vi "HEUI.vi"(0 "LED Update Rate (s)":dbl=0.25 caption="Delay Time (s)", 6 "HEUI_Buttons":T1, 7 "stop":bool, 11 "Error In":errorcluster) -> (5 "HEUI_LEDs":T2, 15 "Error Out":errorcluster)   [LabVIEW 2014]
doc: "This VI controls the high end 2015 VA washer UI board. The VI updates the status of the LEDs every 'LED update rate (s)' number of seconds. The VI allows the user to press buttons and select a cycle."
uses:
  type defs/HEUI_Buttons.ctl
  type defs/HEUI_LEDs.ctl
  Utility/Labview GEA2 Toolkit v2.1/type defs/Data In.ctl
  Utility/Labview GEA2 Toolkit v2.1/type defs/Source_Destination.ctl
  Utility/Labview GEA2 Toolkit v2.1/type defs/ERD Read Data In.ctl
  Utility/Labview GEA2 Toolkit v2.1/type defs/ERD Write Data In.ctl
  type defs/HEUI Switches.ctl
  Utility/Labview GEA2 Toolkit v2.1/library/GEA2_Toolkit.lvlib
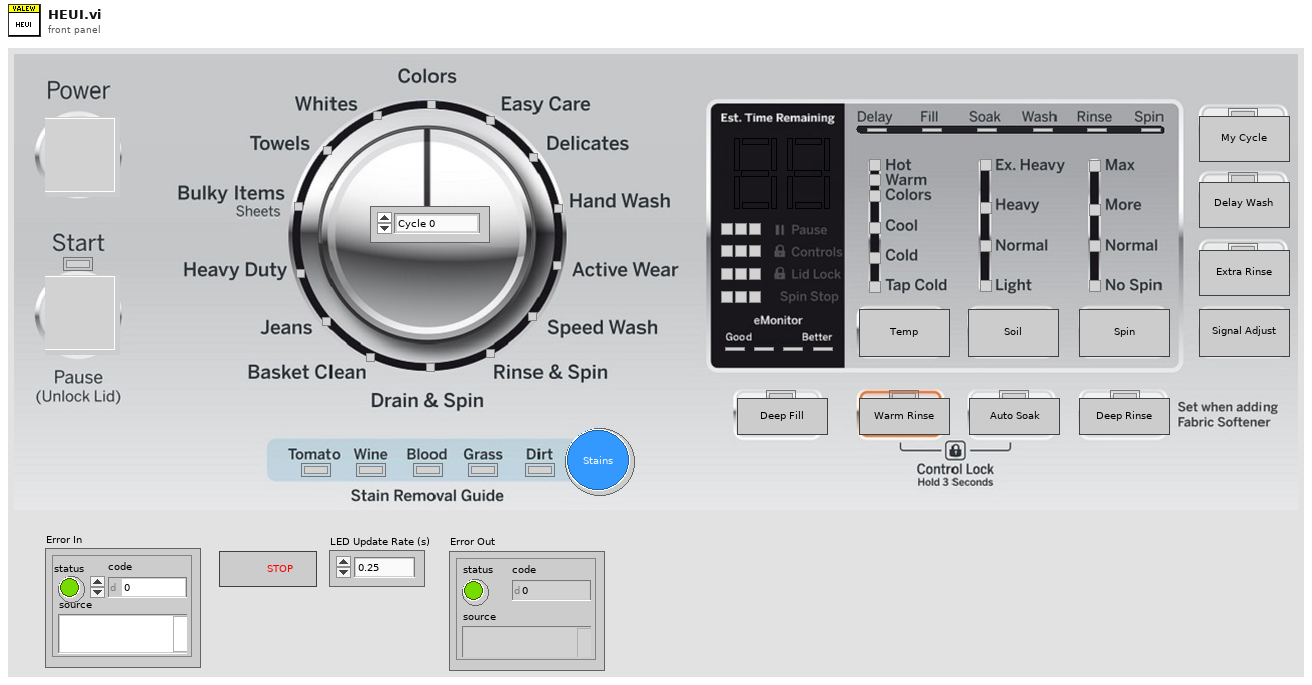
[diagram p1: front panel]
types:
  T1 = typedef "HEUI_Buttons.ctl" = cluster{"SW204 - Signal Adjust":bool, "SW203 - Extra Rinse":bool, "SW201 - My Cycle":bool, "SW202 - Delay Wash":bool, "SW211 - Deep Fill":bool, "SW210 - Warm Rinse":bool, "SW208 - Auto Soak":bool, "SW206 - Deep Rinse":bool, "SW209 - Temp":bool, "SW207 - Soil":bool, "SW205 - Spin":bool, "SW212 - Stains":bool, "Cycle Selection":enum16{"Cycle 0", "Cycle 1", "Cycle 2", "Cycle 3", "Cycle 4", "Cycle 5", "Cycle 6", "Cycle 7", "Cycle 8", "Cycle 9", "Cycle 10", "Cycle 11", "Cycle 12", "Cycle 13"}, "SW213 - Power":bool, "SW214 - Start/Pause":bool}
  T2 = typedef "HEUI_LEDs.ctl" = cluster{"Z101 - Start":bool, "Z103 - Colors":bool, "Z104 - Whites":bool, "Z105 - Towels":bool, "Z106 - Bulky Items":bool, "Z107 - Heavy Duty":bool, "Z108 - Jeans":bool, "Z109 - Basket Clean":bool, "Z110 - Drain and Spin":bool, "Z111 - Rinse and Spin":bool, "Z112 - Speed Wash":bool, "Z113 - Active Wear":bool, "Z114 - Hand Wash":bool, "Z115 - Delicates":bool, "Z116 - Easy Care":bool, "Z117 - Tomato":bool, "Z118 - Wine":bool, "Z119 - Blood":bool, "Z120 - Grass":bool, "Z121 - Dirt":bool, "Z122_MSB_A":bool, "Z123_MSB_B":bool, "Z124_MSB_G":bool, "Z125_MSB_C":bool, "Z126_MSB_D":bool, "Z127_MSB_E":bool, "Z128_MSB_F":bool, "Z129_LSB_A":bool, "Z130_LSB_B":bool, "Z131_LSB_G":bool, "Z132_LSB_C":bool, "Z133_LSB_D":bool, "Z134_LSB_E":bool, "Z135_LSB_F":bool, "Z136 - Pause":bool, "Z137 - Pause":bool, "Z138 - Lock Controls":bool, "Z139 - Lock Controls":bool, "Z140 - Lock Controls":bool, "Z141 - Lid Lock":bool, "Z142 - Lid Lock":bool, "Z143 - Lid Lock":bool, "Z144 - Good":bool, "Z145":bool, "Z146":bool, "Z147 - Better":bool, "Z148 - Delay":bool, "Z149 - Fill":bool, "Z150 - Soak":bool, "Z151 - Wash":bool, "Z152 - Rinse":bool, "Z153 - Spin":bool, "Z154 - Hot":bool, "Z155 - Warm":bool, "Z156 - Colors":bool, "Z157 - Cool":bool, "Z158 - Cold":bool, "Z159 - Tap Cold":bool, "Z160 - Extra Heavy":bool, "Z161 - Heavy":bool, "Z162 - Normal":bool, "Z163 - Light":bool, "Z164 - Max Spin":bool, "Z165 - More Spin":bool, "Z166 - Normal Spin":bool, "Z167 - No Spin":bool, "Z168 - Extra Rinse":bool, "Z170 - Deep Rinse":bool, "Z171 - Auto Soak":bool, "Z172 - Warm Rinse":bool, "Z173 - Deep Fill":bool, "Z174 - My Cycles":bool, "Z175 - Delay Wash":bool, "Z176 - Spin Stop":bool, "Z177 - Spin Stop":bool, "Z178 - Spin Stop":bool, "Z179 - Pause":bool, "Z109":bool, "Z110":bool, "Z123":bool, "Z124":bool, "Z140":bool, "Unused0":bool, "Unused1":bool, "Unused2":bool, "Unused3":bool, "Channel_Off":bool, "Channel_Cycle_Unmapped":bool}
  T3 = typedef "GEA2_Toolkit.lvlib/ERD Write Data In.ctl" = cluster{"ERD Number":u16, "Data Type":enum16{"string", "boolean", "uint8_t", "uint16_t", "uint32_t"}, "Data":string}
  T4 = typedef "GEA2_Toolkit.lvlib/ERD Read Data In.ctl" = cluster{"ERD Number":u16, "Data Type":enum16{"string", "boolean", "uint8_t", "uint16_t", "uint32_t", "uint64_t"}}
  T5 = typedef "GEA2_Toolkit.lvlib/Source_Destination.ctl" = cluster{"Source":u8, "Destination":u8}
  T6 = typedef "GEA2_Toolkit.lvlib/Data In.ctl" = cluster{"Source":u8, "Destination":u8, "Command":u8, "Message":string}
  T7 = typedef "HEUI Switches.ctl" = enum16{"Switch Off", "SW201 - My Cycle", "SW202 - Delay Wash", "SW203 - Extra Rinse", "SW204 - Signal Adjust", "SW205 - Spin", "SW206 - Deep Rinse", "SW207 - Soil", "SW208 - Auto Soak", "SW209 - Temp", "SW210 - Warm Rinse", "SW211 - Deep Fill", "SW212 - Stains", "SW213 - Power", "SW214 - Start/Pause", "SW215", "SW216"}
  T8 = enum16{"string", "boolean", "uint8_t", "uint16_t", "uint32_t"}
  T9 = enum16{"Cycle 0", "Cycle 1", "Cycle 2", "Cycle 3", "Cycle 4", "Cycle 5", "Cycle 6", "Cycle 7", "Cycle 8", "Cycle 9", "Cycle 10", "Cycle 11", "Cycle 12", "Cycle 13"}
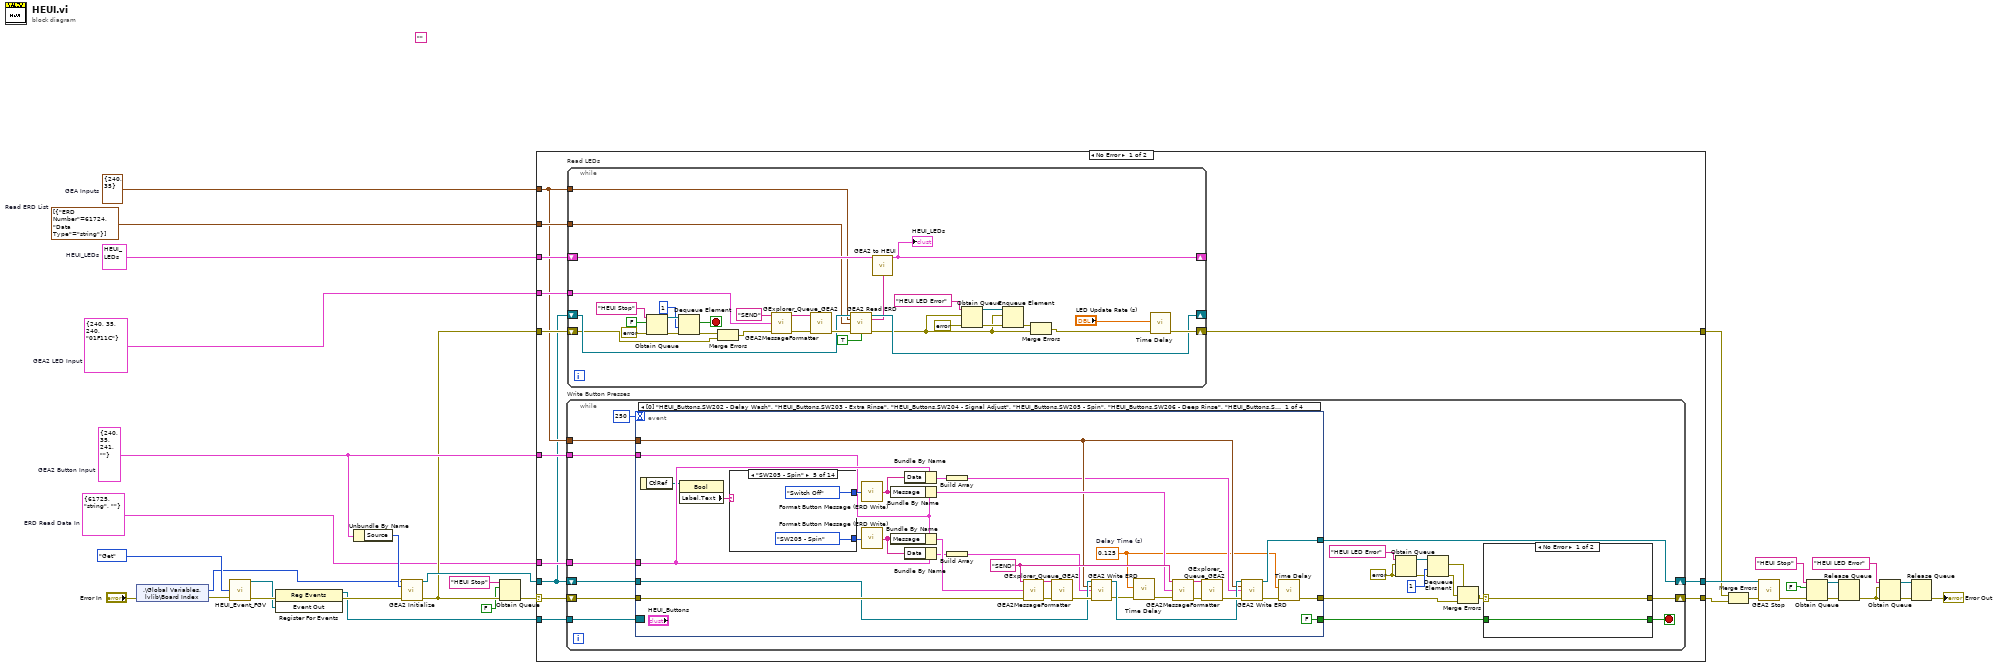
[diagram p0: block diagram]
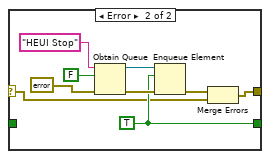
[diagram p2: hidden frame]
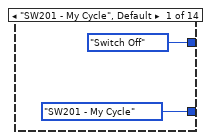
[diagram p3: hidden frame]
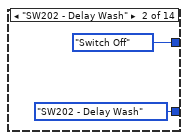
[diagram p4: hidden frame]
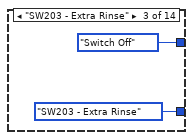
[diagram p5: hidden frame]
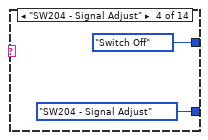
[diagram p6: hidden frame]
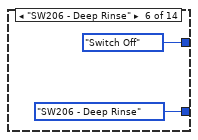
[diagram p7: hidden frame]
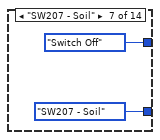
[diagram p8: hidden frame]
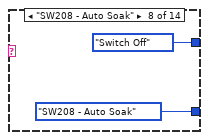
[diagram p9: hidden frame]
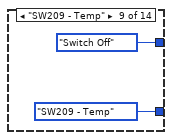
[diagram p10: hidden frame]
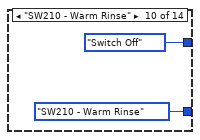
[diagram p11: hidden frame]
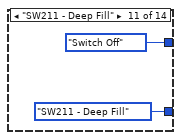
[diagram p12: hidden frame]
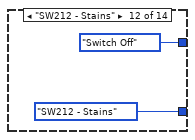
[diagram p13: hidden frame]
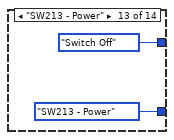
[diagram p14: hidden frame]
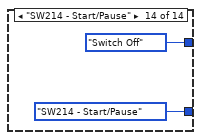
[diagram p15: hidden frame]
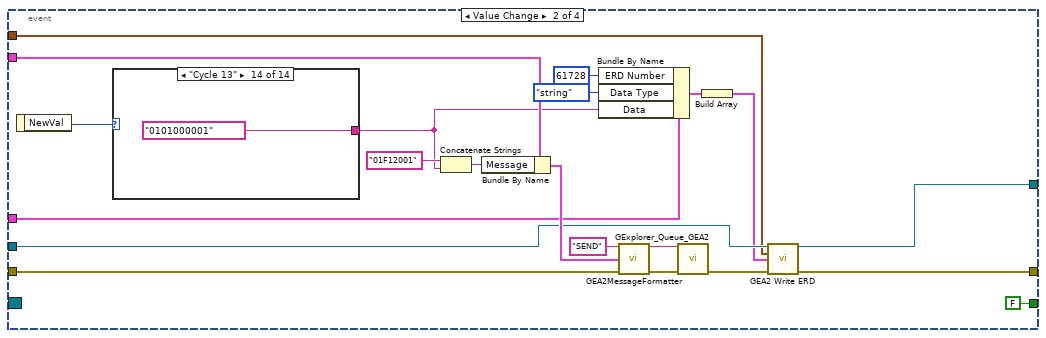
[diagram p16: hidden frame]
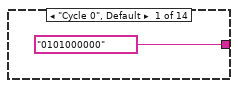
[diagram p17: hidden frame]
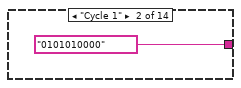
[diagram p18: hidden frame]
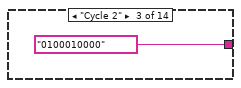
[diagram p19: hidden frame]
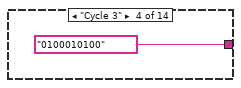
[diagram p20: hidden frame]
diagram:
  w15 = T3 {"ERD Number"=61725, "Data Type"=enum."string", "Data"=""}  # ERD Read Data In
  w17 = T4[] [{"ERD Number"=61724, "Data Type"=enum."string"}]  # Read ERD List
  w16 = T5 {"Source"=240, "Destination"=35}  # GEA Inputs
  w27 = T6 {"Source"=240, "Destination"=35, "Command"=240, "Message"="01F11C"}  # GEA2 LED Input
  w28 = T2 {"Z101 - Start"=FALSE, "Z103 - Colors"=FALSE, "Z104 - Whites"=FALSE, "Z105 - Towels"=FALSE, "Z106 - Bulky Items"=FALSE, "Z107 - Heavy Duty"=FALSE, "Z108 - Jeans"=FALSE, "Z109 - Basket Clean"=FALSE, "Z110 - Drain and Spin"=FALSE, "Z111 - Rinse and Spin"=FALSE, "Z112 - Speed Wash"=FALSE, "Z113 - Active Wear"=FALSE, "Z114 - Hand Wash"=FALSE, "Z115 - Delicates"=FALSE, "Z116 - Easy Care"=FALSE, "Z117 - Tomato"=FALSE, "Z118 - Wine"=FALSE, "Z119 - Blood"=FALSE, "Z120 - Grass"=FALSE, "Z121 - Dirt"=FALSE, "Z122_MSB_A"=FALSE, "Z123_MSB_B"=FALSE, "Z124_MSB_G"=FALSE, "Z125_MSB_C"=FALSE, "Z126_MSB_D"=FALSE, "Z127_MSB_E"=FALSE, "Z128_MSB_F"=FALSE, "Z129_LSB_A"=FALSE, "Z130_LSB_B"=FALSE, "Z131_LSB_G"=FALSE, "Z132_LSB_C"=FALSE, "Z133_LSB_D"=FALSE, "Z134_LSB_E"=FALSE, "Z135_LSB_F"=FALSE, "Z136 - Pause"=FALSE, "Z137 - Pause"=FALSE, "Z138 - Lock Controls"=FALSE, "Z139 - Lock Controls"=FALSE, "Z140 - Lock Controls"=FALSE, "Z141 - Lid Lock"=FALSE, "Z142 - Lid Lock"=FALSE, "Z143 - Lid Lock"=FALSE, "Z144 - Good"=FALSE, "Z145"=FALSE, "Z146"=FALSE, "Z147 - Better"=FALSE, "Z148 - Delay"=FALSE, "Z149 - Fill"=FALSE, "Z150 - Soak"=FALSE, "Z151 - Wash"=FALSE, "Z152 - Rinse"=FALSE, "Z153 - Spin"=FALSE, "Z154 - Hot"=FALSE, "Z155 - Warm"=FALSE, "Z156 - Colors"=FALSE, "Z157 - Cool"=FALSE, "Z158 - Cold"=FALSE, "Z159 - Tap Cold"=FALSE, "Z160 - Extra Heavy"=FALSE, "Z161 - Heavy"=FALSE, "Z162 - Normal"=FALSE, "Z163 - Light"=FALSE, "Z164 - Max Spin"=FALSE, "Z165 - More Spin"=FALSE, "Z166 - Normal Spin"=FALSE, "Z167 - No Spin"=FALSE, "Z168 - Extra Rinse"=FALSE, "Z170 - Deep Rinse"=FALSE, "Z171 - Auto Soak"=FALSE, "Z172 - Warm Rinse"=FALSE, "Z173 - Deep Fill"=FALSE, "Z174 - My Cycles"=FALSE, "Z175 - Delay Wash"=FALSE, "Z176 - Spin Stop"=FALSE, "Z177 - Spin Stop"=FALSE, "Z178 - Spin Stop"=FALSE, "Z179 - Pause"=FALSE, "Z109"=FALSE, "Z110"=FALSE, "Z123"=FALSE, "Z124"=FALSE, "Z140"=FALSE, "Unused0"=FALSE, "Unused1"=FALSE, "Unused2"=FALSE, "Unused3"=FALSE, "Channel_Off"=FALSE, "Channel_Cycle_Unmapped"=FALSE}  # HEUI_LEDs
  w26 = T6 {"Source"=240, "Destination"=35, "Command"=241, "Message"=""}  # GEA2 Button Input
  (unwired) ""
  n1 = shared-variable ".\\Global Variables.lvlib\\Board Index"(error in="Error In") -> (w1:i32, error out=w2:errorcluster)
  n2 = call "HEUI_Event_FGV.vi"("Action"=enum16{"Get", "Set"}."Get", "Error In"=w2) -> ("Event Out"=w4:refnum<user-event>, "Error Out"=w5:errorcluster)  [unwired: 12 in]
  n3 = register-events(error in=w5, w4) -> (reference out=w7:refnum<event-registration>, error out=w8:errorcluster)  [unwired: 1 in]
  n4 = Unbundle By Name(w26) -> ("Source"=w33:u8)
  n5 = call "GEA2 Initialize.vi"("Board Index"=w1, "Source Address"=w33, "error in"=w8) -> ("GEA2 Reference Out"=w32:refnum<k24>, "error out"=w24:errorcluster)  [unwired: 10 in, 1 out]
  n6 = Obtain Queue(name (unnamed)="HEUI Stop", element data type=FALSE ("stop"), error in (no error)=w24) -> (error out=w14:errorcluster)  [unwired: 2 in, 2 out]
  n7 = case shown="No Error" w14 {
    selector: w14 -> [w36 w238]
    tunnel: [w47 w236] -> w34
    tunnel: w32 -> [w37 w236]
    tunnel: [w46 errorcluster {"status"=FALSE, "code"=0, "source"=""} ("error out")] -> w31
    tunnel: [w45 w238] -> w30
    tunnel: w28 -> [w44 _]
    tunnel: w27 -> [w43 _]
    tunnel: w26 -> [w42 _]
    tunnel: w24 -> [w41 _]
    tunnel: w17 -> [w40 _]
    tunnel: w16 -> [w39 _]
    tunnel: w15 -> [w38 _]
    tunnel: w7 -> [w35 _]
    frame No Error {
      n8 = while "Write Button Presses" {
        shift-right: [w93] -> w45
        shift-left: w36 -> [w99]
        shift-right: [w97] -> w47
        shift-left: w37 -> [w98]
        tunnel: w42 -> [w96]
        tunnel: w39 -> [w95]
        tunnel: w38 -> [w94]
        tunnel: w35 -> [w80]
        stop <- w91 stop-if-true
        w85 = errorcluster {"status"=FALSE, "code"=0, "source"=""} ("error in (no error)")
        n9 = event shown="[0] \"HEUI_Buttons.SW202 - Delay Wash\", \"HEUI_Buttons.SW203 - Extra Rinse\", \"HEUI_Buttons.SW204 - Signal Adjust\", \"HEUI_Buttons.SW205 - Spin\", \"HEUI_Buttons.SW206 - Deep Rinse\", \"HEUI_Buttons.SW207 - Soil\", \"HEUI_Buttons.SW208 - Auto Soak\", \"HEUI_Buttons.SW209 - Temp\", \"HEUI_Buttons.SW210 - Warm Rinse\", \"HEUI_Buttons.SW211 - Deep Fill\", \"HEUI_Buttons.SW212 - Stains\", \"HEUI_Buttons.SW213 - Power\", \"HEUI_Buttons.SW214 - Start/Pause\", \"HEUI_Buttons.SW201 - My Cycle\": Value Change" {
          selector: w80 -> [_ _ _ _]
          dyn-events: _ -> [_ _ _ _]
          timeout: 250 -> [_ _ _ _]
          tunnel: [w116 w183 w231 w234] -> w83
          tunnel: w99 -> [w140 w191 w212 w234]
          tunnel: w98 -> [w131 w182 w208 w235]
          tunnel: [w129 w181 w206 w235] -> w97
          tunnel: [FALSE ("stop") FALSE ("stop") w230 FALSE ("stop")] -> w92
          tunnel: w96 -> [w113 w190 w214 _]
          tunnel: w95 -> [w127 w180 w207 _]
          tunnel: w94 -> [w122 w179 w210 _]
          event Value Change {
            w112 = 0.125  # Delay Time (s)
            w138 = "SEND" ("Prefix(Send/Recv)")
            n10 = event-data() -> ("CtlRef"=w115:refnum<vi>)  [unwired: 1 in]
            n11 = property class="Bool"(reference=w115) -> ("Label.Text"=w114:string)  [unwired: 1 in, 2 out]
            n12 = case shown="\"SW205 - Spin\"" w114 {
              tunnel: [HEUI_Switches."SW201 - My Cycle" ("Switch") HEUI_Switches."SW202 - Delay Wash" ("Switch") HEUI_Switches."SW203 - Extra Rinse" ("Switch") HEUI_Switches."SW204 - Signal Adjust" ("Switch") HEUI_Switches."SW205 - Spin" ("Switch") HEUI_Switches."SW206 - Deep Rinse" ("Switch") HEUI_Switches."SW207 - Soil" ("Switch") HEUI_Switches."SW208 - Auto Soak" ("Switch") HEUI_Switches."SW209 - Temp" ("Switch") HEUI_Switches."SW210 - Warm Rinse" ("Switch") HEUI_Switches."SW211 - Deep Fill" ("Switch") HEUI_Switches."SW212 - Stains" ("Switch") HEUI_Switches."SW213 - Power" ("Switch") HEUI_Switches."SW214 - Start/Pause" ("Switch")] -> w142
              tunnel: [HEUI_Switches."Switch Off" ("Switch") HEUI_Switches."Switch Off" ("Switch") HEUI_Switches."Switch Off" ("Switch") HEUI_Switches."Switch Off" ("Switch") HEUI_Switches."Switch Off" ("Switch") HEUI_Switches."Switch Off" ("Switch") HEUI_Switches."Switch Off" ("Switch") HEUI_Switches."Switch Off" ("Switch") HEUI_Switches."Switch Off" ("Switch") HEUI_Switches."Switch Off" ("Switch") HEUI_Switches."Switch Off" ("Switch") HEUI_Switches."Switch Off" ("Switch") HEUI_Switches."Switch Off" ("Switch") HEUI_Switches."Switch Off" ("Switch")] -> w133
              frame "SW201 - My Cycle", Default {
              }
              frame "SW202 - Delay Wash" {
              }
              frame "SW203 - Extra Rinse" {
              }
              frame "SW204 - Signal Adjust" {
              }
              frame "SW205 - Spin" {
              }
              frame "SW206 - Deep Rinse" {
              }
              frame "SW207 - Soil" {
              }
              frame "SW208 - Auto Soak" {
              }
              frame "SW209 - Temp" {
              }
              frame "SW210 - Warm Rinse" {
              }
              frame "SW211 - Deep Fill" {
              }
              frame "SW212 - Stains" {
              }
              frame "SW213 - Power" {
              }
              frame "SW214 - Start/Pause" {
              }
            }
            n13 = call "Format Button Message (ERD Write).vi"("Switch"=w133) -> ("Switch Message"=w126:string)  [unwired: 14 in]
            n14 = call "Format Button Message (ERD Write).vi"("Switch"=w142) -> ("Switch Message"=w120:string)  [unwired: 14 in]
            n15 = Bundle By Name(cluster=w113, "Message"=w126) -> (w134:T6)
            n16 = Bundle By Name(cluster=w113, "Message"=w120) -> (w135:T6)
            n17 = Bundle By Name(cluster=w122, "Data"=w126) -> (w125:T3)
            n18 = Bundle By Name(cluster=w122, "Data"=w120) -> (w123:T3)
            n19 = Build Array(w125) -> (w124:T3[])
            n20 = Build Array(w123) -> (w121:T3[])
            n21 = call "GEA2MessageFormatter.vi"("Prefix(Send/Recv)"=w138, "GEA2 Data In"=w135, "Error In"=w140) -> ("Output String"=w137:string, "Error Out"=w141:errorcluster)  [unwired: 11 in]
            n22 = call "GExplorer_Queue_GEA2.vi"("Output String"=w137, "error in (no error)"=w141) -> ("error out"=w132:errorcluster)  [unwired: 13 in]
            n23 = call "GEA2 Write ERD.vi"("GEA2 Reference In"=w131, "GEA Inputs"=w127, "Write ERD List"=w121, "Error In"=w132) -> ("GEA2 Reference Out"=w128:refnum<k24>, "Error Out"=w119:errorcluster)  [unwired: 9 in, 1 out]
            n24 = call "Time Delay"("error in (no error)"=w119, "Delay Time (s)"=w112) -> ("error out"=w118:errorcluster)  [unwired: 9 in]
            n25 = call "GEA2MessageFormatter.vi"("Prefix(Send/Recv)"=w138, "GEA2 Data In"=w134, "Error In"=w118) -> ("Output String"=w136:string, "Error Out"=w139:errorcluster)  [unwired: 11 in]
            n26 = call "GExplorer_Queue_GEA2.vi"("Output String"=w136, "error in (no error)"=w139) -> ("error out"=w130:errorcluster)  [unwired: 13 in]
            n27 = call "GEA2 Write ERD.vi"("GEA2 Reference In"=w128, "GEA Inputs"=w127, "Write ERD List"=w124, "Error In"=w130) -> ("GEA2 Reference Out"=w129:refnum<k24>, "Error Out"=w117:errorcluster)  [unwired: 9 in, 1 out]
            n28 = call "Time Delay"("error in (no error)"=w117, "Delay Time (s)"=w112) -> ("error out"=w116:errorcluster)  [unwired: 9 in]
          }
          event Value Change {
            n29 = event-data() -> ("NewVal"=w174:T9)  [unwired: 1 in]
            n30 = case shown="\"Cycle 13\"" w174 {
              tunnel: ["0101000000" "0101010000" "0100010000" "0100010100" "0101010100" "0101000100" "0100000100" "0100000101" "0101000101" "0101010101" "0100010101" "0100010001" "0101010001" "0101000001"] -> w172
              frame "Cycle 0", Default {
              }
              frame "Cycle 1" {
              }
              frame "Cycle 2" {
              }
              frame "Cycle 3" {
              }
              frame "Cycle 4" {
              }
              frame "Cycle 5" {
              }
              frame "Cycle 6" {
              }
              frame "Cycle 7" {
              }
              frame "Cycle 8" {
              }
              frame "Cycle 9" {
              }
              frame "Cycle 10" {
              }
              frame "Cycle 11" {
              }
              frame "Cycle 12" {
              }
              frame "Cycle 13" {
              }
            }
            n31 = Concatenate Strings("01F12001" ("string"), w172) -> (w173:string)
            n32 = Bundle By Name(cluster=w190, "Message"=w173) -> (w186:T6)
            n33 = Bundle By Name(cluster=w179, "ERD Number"=u16 61728, "Data Type"=T8."string", "Data"=w172) -> (w176:T3)
            n34 = call "GEA2MessageFormatter.vi"("Prefix(Send/Recv)"="SEND", "GEA2 Data In"=w186, "Error In"=w191) -> ("Output String"=w185:string, "Error Out"=w189:errorcluster)  [unwired: 11 in]
            n35 = call "GExplorer_Queue_GEA2.vi"("Output String"=w185, "error in (no error)"=w189) -> ("error out"=w184:errorcluster)  [unwired: 13 in]
            n36 = Build Array(w176) -> (w175:T3[])
            n37 = call "GEA2 Write ERD.vi"("GEA2 Reference In"=w182, "GEA Inputs"=w180, "Write ERD List"=w175, "Error In"=w184) -> ("GEA2 Reference Out"=w181:refnum<k24>, "Error Out"=w183:errorcluster)  [unwired: 9 in, 1 out]
          }
          event "stop": Value Change; Panel Close; User Event {
            w213 = "0000000000" ("string")
            w230 = TRUE ("stop")
            n38 = event-data() -> ()  [unwired: 1 in, 1 out]
            n39 = Concatenate Strings("01F12001" ("string"), w213) -> (w215:string)
            n40 = Bundle By Name(cluster=w214, "Message"=w215) -> (w221:T6)
            n41 = Bundle By Name(cluster=w210, "ERD Number"=u16 61728, "Data Type"=T8."string", "Data"=w213) -> (w216:T3)
            n42 = call "GEA2MessageFormatter.vi"("Prefix(Send/Recv)"="SEND", "GEA2 Data In"=w221, "Error In"=w212) -> ("Output String"=w220:string, "Error Out"=w224:errorcluster)  [unwired: 11 in]
            n43 = call "GExplorer_Queue_GEA2.vi"("Output String"=w220, "error in (no error)"=w224) -> ("error out"=w219:errorcluster)  [unwired: 13 in]
            n44 = Build Array(w216) -> (w209:T3[])
            n45 = call "GEA2 Write ERD.vi"("GEA2 Reference In"=w208, "GEA Inputs"=w207, "Write ERD List"=w209, "Error In"=w219) -> ("GEA2 Reference Out"=w206:refnum<k24>, "Error Out"=w211:errorcluster)  [unwired: 9 in, 1 out]
            n46 = control-ref of="This VI"() -> (w232:refnum<vi>)
            n47 = invoke class="VI" method="FP.Close"(reference=w232, error in=w211) -> (error out=w229:errorcluster)  [unwired: 1 in, 2 out]
            n48 = Obtain Queue(name (unnamed)="HEUI Stop", element data type=FALSE ("stop"), error in (no error)=w229) -> (queue out=w227:refnum<queue>, error out=w228:errorcluster)  [unwired: 2 in, 1 out]
            n49 = Enqueue Element(queue=w227, element=w230, error in (no error)=w228) -> (error out=w231:errorcluster)  [unwired: 1 in, 2 out]
          }
          event Timeout {
            n50 = event-data() -> ()  [unwired: 1 in, 3 out]
          }
        }
        n51 = Obtain Queue(name (unnamed)="HEUI LED Error", element data type=w85, error in (no error)=w85) -> (queue out=w87:refnum<queue>, error out=w88:errorcluster)  [unwired: 2 in, 1 out]
        n52 = Dequeue Element(queue=w87, timeout in ms (-1)=1, error in (no error)=w88) -> (element=w81:errorcluster, error out=w82:errorcluster)  [unwired: 2 out]
        n53 = Merge Errors(w81, w82, w83) -> (w86:errorcluster)
        n54 = case shown="No Error" w86 {
          selector: w86 -> [w101 w103]
          tunnel: [w101 w105] -> w93
          tunnel: w92 -> [w100 _]
          tunnel: [w100 w106] -> w91
          frame No Error {
          }
          frame Error {
            w106 = TRUE ("stop")
            n55 = Obtain Queue(name (unnamed)="HEUI Stop", element data type=FALSE ("stop"), error in (no error)=errorcluster {"status"=FALSE, "code"=0, "source"=""}) -> (queue out=w109:refnum<queue>, error out=w110:errorcluster)  [unwired: 2 in, 1 out]
            n56 = Enqueue Element(queue=w109, element=w106, error in (no error)=w110) -> (error out=w104:errorcluster)  [unwired: 1 in, 2 out]
            n57 = Merge Errors(w104, w103) -> (w105:errorcluster)
          }
        }
      }
      n58 = while "Read LEDs" {
        shift-right: [w77] -> w46
        shift-left: w41 -> [w48]
        shift-right: [w64] -> _
        shift-left: w37 -> [w63]
        tunnel: w43 -> [w72]
        tunnel: w39 -> [w62]
        tunnel: w40 -> [w61]
        shift-right: [w79] -> _
        shift-left: w44 -> [w78]
        stop <- w71 stop-if-true
        n59 = Obtain Queue(name (unnamed)="HEUI Stop", element data type=FALSE ("stop"), error in (no error)=errorcluster {"status"=FALSE, "code"=0, "source"=""}) -> (queue out=w70:refnum<queue>, error out=w69:errorcluster)  [unwired: 2 in, 1 out]
        n60 = Dequeue Element(queue=w70, timeout in ms (-1)=1, error in (no error)=w69) -> (element=w71:bool, error out=w51:errorcluster)  [unwired: 2 out]
        n61 = Merge Errors(w51, w48) -> (w50:errorcluster)
        n62 = call "GEA2MessageFormatter.vi"("Prefix(Send/Recv)"="SEND", "GEA2 Data In"=w72, "Error In"=w50) -> ("Output String"=w74:string, "Error Out"=w73:errorcluster)  [unwired: 11 in]
        n63 = call "GExplorer_Queue_GEA2.vi"("Output String"=w74, "error in (no error)"=w73) -> ("error out"=w65:errorcluster)  [unwired: 13 in]
        n64 = call "GEA2 Read ERD.vi"("GEA2 Reference In"=w63, "GEA Inputs"=w62, "Read ERD List"=w61, "Error In"=w65, "Verify ERD Response?"=TRUE) -> ("GEA2 Reference Out"=w64:refnum<k24>, "Raw Data Out"=w60:string, "Error Out"=w54:errorcluster)  [unwired: 7 in, 1 out]
        n65 = call "GEA2 to HEUI.vi"("HEUI_LEDs_In"=w78, "Raw Data In"=w60) -> ("HEUI_LEDs_Out"=w79:T2)  [unwired: 13 in]
        "HEUI_LEDs" <- w79
        n66 = Obtain Queue(name (unnamed)="HEUI LED Error", element data type=w54, error in (no error)=errorcluster {"status"=FALSE, "code"=0, "source"=""}) -> (queue out=w57:refnum<queue>, error out=w56:errorcluster)  [unwired: 2 in, 1 out]
        n67 = Enqueue Element(queue=w57, element=w54, error in (no error)=w56) -> (error out=w55:errorcluster)  [unwired: 1 in, 2 out]
        n68 = Merge Errors(w55, w54) -> (w53:errorcluster)
        n69 = call "Time Delay"("error in (no error)"=w53, "Delay Time (s)"="LED Update Rate (s)") -> ("error out"=w77:errorcluster)  [unwired: 9 in]
      }
    }
    frame Error {
    }
  }
  n70 = Merge Errors(w31, w30) -> (w29:errorcluster)
  n71 = call "GEA2 Stop.vi"("GEA2 Reference In"=w34, "Error In"=w29) -> ("Error Out"=w18:errorcluster)  [unwired: 13 in]
  n72 = Obtain Queue(name (unnamed)="HEUI Stop", element data type=FALSE ("stop"), error in (no error)=w18) -> (queue out=w19:refnum<queue>, error out=w20:errorcluster)  [unwired: 2 in, 1 out]
  n73 = Release Queue(queue=w19, error in (no error)=w20) -> (error out=w10:errorcluster)  [unwired: 1 in, 2 out]
  n74 = Obtain Queue(name (unnamed)="HEUI LED Error", element data type=w10, error in (no error)=w10) -> (queue out=w13:refnum<queue>, error out=w12:errorcluster)  [unwired: 2 in, 1 out]
  n75 = Release Queue(queue=w13, error in (no error)=w12) -> (error out=→"Error Out":errorcluster)  [unwired: 1 in, 2 out]
